vi "RT FIFO Variables - local.vi"() -> ()   [LabVIEW 2017]
doc: "Uses RT FIFO-enabled shared variables to communicate data between loops of different priorities without impacting determinism."
uses:
  <vilib>/Platform/TimedLoop/XDataNode/timing_clust.ctl
  <vilib>/Platform/TimedLoop/XDataNode/nitl_modes.ctl
  <vilib>/Platform/TimedLoop/XDataNode/wakeup.ctl
  <vilib>/platform/TimedLoop/XDataNode/XDataNode.xnode
  <vilib>/Platform/TimedLoop/XDataNode/XDNodeRunTimeDep.lvlib
panel:
  in  "Amplitude":dbl(slide)=5.0 scale=0.0..10.0
  in  "Stop":bool
  out "Result Data":dbl(graph)
  # "Overview: Uses RT FIFO-enabled shared variables to communicate data between loops of different priorities without impacting determinism.\nRequirements: LabVIEW Real-Time Module\nInstructions:\n1. In Measurement & Automation Explorer, ensure that LabVIEW Real-Time and the Network Variable Engine are installed on your RT target.\n2. From the Project Explorer window, set the IP address of your RT target.\n3. Run the VI.\n4. Adjust the Amplitude slider, which will update Result Data chart. \n5. Click the Stop button."
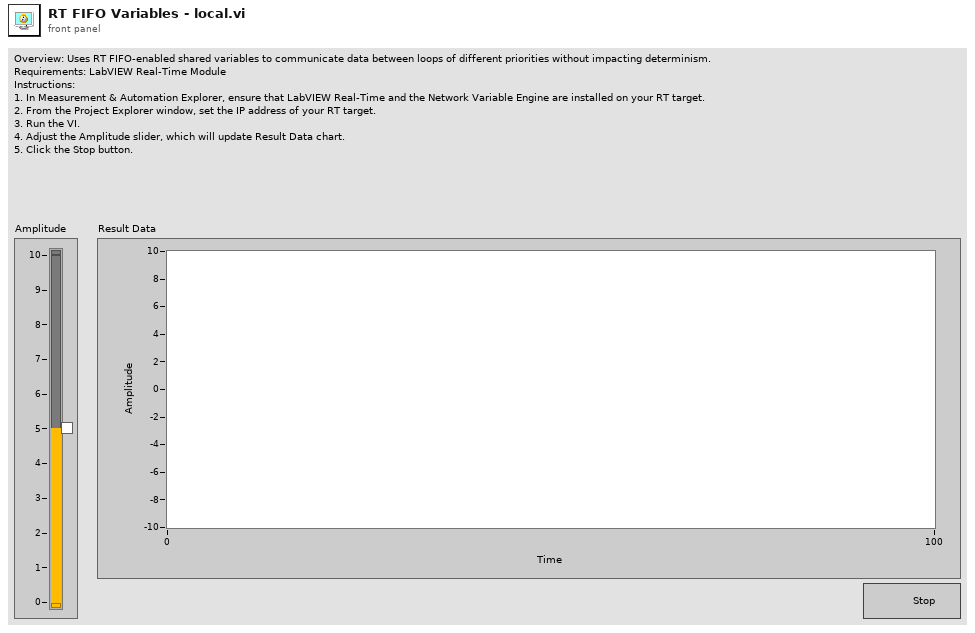
[diagram p1: front panel]
types:
  T1 = typedef "XDNodeRunTimeDep.lvlib/timing_clust.ctl" = cluster{"Expected End [f-1]":u64, "Actual End [f-1]":u64, "Finished Late? [f-1]":bool, "Expected End [i-1]":u64, "Actual End [i-1]":u64, "Finished Late? [i-1]":bool, "Expected Start [i]":u64, "Actual Start [i]":u64, "Expected Start [f]":u64, "Actual Start [f]":u64, "Source Name":string, "Structure Name":string, "Period":i64, "Deadline":i64, "Offset":i64, "Start":i64, "Priority":i32, "Timeout":i32, "Mode":T2, "Wakeup Reason":T3, "Error":errorcluster, "Source Type":string, "Secondary Source Type":string, "Global End Time":u64, "Global Start Time":u64, "Frame Duration":u64, "Iteration Duration":u64, "Assigned CPU":i32, "I/O Scan Engine Mode":u32}
  T2 = typedef "XDNodeRunTimeDep.lvlib/nitl_modes.ctl" = enum32{"No Change", "Process missed periods, maintain original phase", "Discard missed periods, maintain original phase", "Process missed periods, ignore original phase", "Discard missed periods, ignore original phase"}
  T3 = typedef "XDNodeRunTimeDep.lvlib/wakeup.ctl" = enum32{"Normal", "Aborted", "Asynchronous wakeup", "Timing source error", "Timed loop error", "Timeout"}
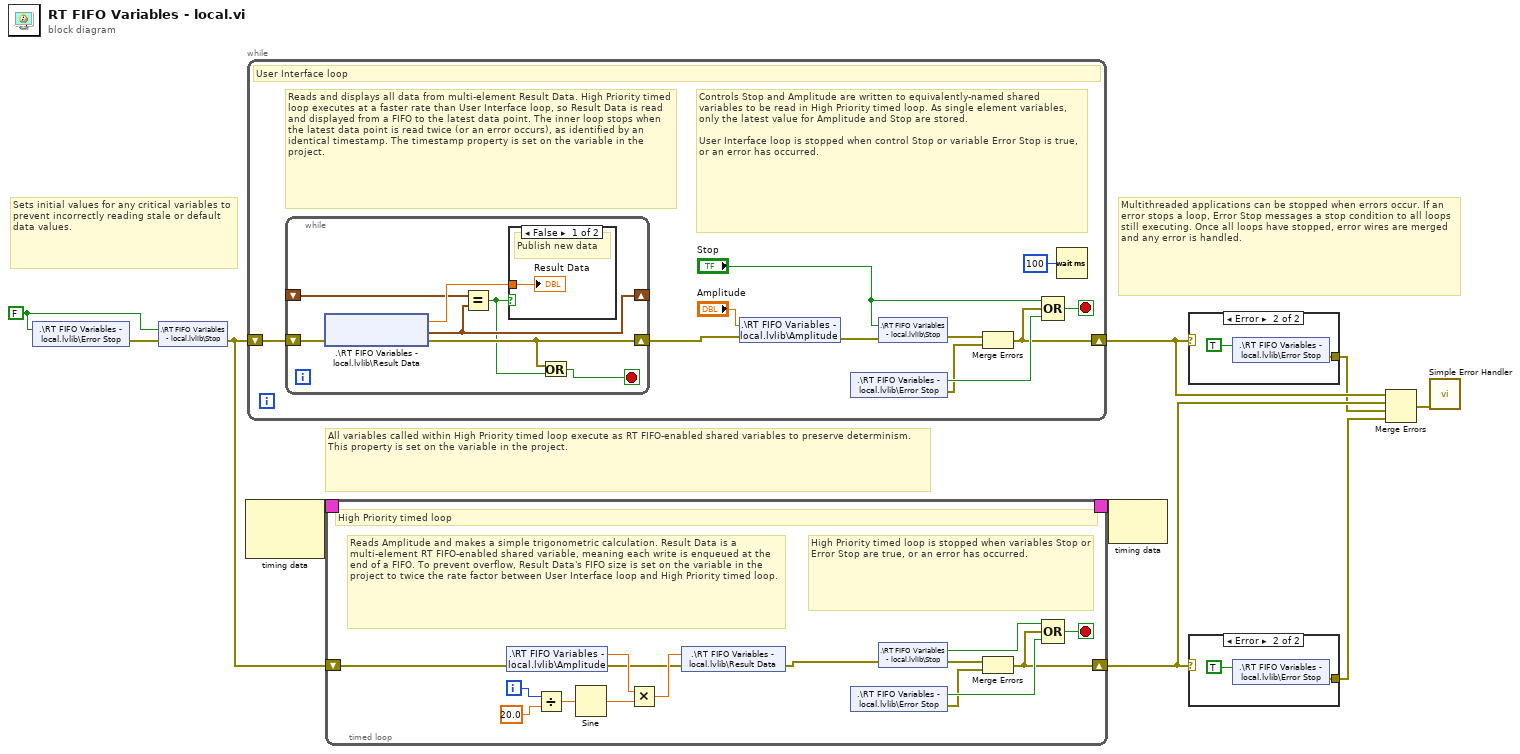
[diagram p0: block diagram]
diagram:
  w6 = FALSE ("Stop")
  # "All variables called within High Priority timed loop execute as RT FIFO-enabled shared variables to preserve determinism. This property is set on the variable in the project."
  # "Multithreaded applications can be stopped when errors occur. If an error stops a loop, Error Stop messages a stop condition to all loops still executing. Once all loops have stopped, error wires are merged and any error is handled."
  # "Sets initial values for any critical variables to prevent incorrectly reading stale or default data values."
  n1 = shared-variable ".\\RT FIFO Variables - local.lvlib\\Error Stop"(w6) -> (error out=w7:errorcluster)  [unwired: 1 in]
  n2 = shared-variable ".\\RT FIFO Variables - local.lvlib\\Stop"(w6, error in=w7) -> (error out=w8:errorcluster)
  n3 = node-c288() -> (w10:T1)  [unwired: 1 in, 1 out]
  n4 = while "User Interface loop" {
    shift-right: [w12] -> w4
    shift-left: w8 -> [w20]
    stop <- w21 stop-if-true
    # "Controls Stop and Amplitude are written to equivalently-named shared variables to be read in High Priority timed loop. As single element variables, only the latest value for Amplitude and Stop are stored.\n\nUser Interface loop is stopped when control Stop or variable Error Stop is true, or an error has occurred."
    # "Reads and displays all data from multi-element Result Data. High Priority timed loop executes at a faster rate than User Interface loop, so Result Data is read and displayed from a FIFO to the latest data point. The inner loop stops when the latest data point is read twice (or an error occurs), as identified by an identical timestamp. The timestamp property is set on the variable in the project."
    # "User Interface loop"
    n5 = while {
      shift-right: [w26] -> _
      shift-left: _ -> [w25]
      shift-right: [w24] -> w18
      shift-left: w20 -> [w28]
      stop <- w22 stop-if-true
      n6 = shared-variable ".\\RT FIFO Variables - local.lvlib\\Result Data"(error in=w28) -> (w27:dbl, error out=w24:errorcluster, w26:timestamp)
      n7 = Equal?(x=w25, y=w26) -> (x = y?=w23:bool)
      n8 = case shown="False" w23 {
        tunnel: w27 -> [w29 _]
        frame False {
          # "Publish new data"
          "Result Data" <- w29
        }
        frame True {
          # "No new data"
        }
      }
      n9 = Or(x=w24, y=w23) -> (x .or. y?=w22:bool)
    }
    n10 = shared-variable ".\\RT FIFO Variables - local.lvlib\\Amplitude"("Amplitude", error in=w18) -> (error out=w19:errorcluster)
    n11 = shared-variable ".\\RT FIFO Variables - local.lvlib\\Error Stop"() -> (w14:bool, error out=w11:errorcluster)  [unwired: 1 in]
    n12 = shared-variable ".\\RT FIFO Variables - local.lvlib\\Stop"("Stop", error in=w19) -> (error out=w13:errorcluster)
    n13 = Merge Errors(w13, w11) -> (w12:errorcluster)
    n14 = Compound Arithmetic op=OR("Stop", w12, w14) -> (w21:bool)
    n15 = Wait (ms)(milliseconds to wait=u32 100 ("millisecond multiple")) -> ()  [unwired: 1 out]
  }
  n16 = timed-loop "High Priority timed loop" {
    timing: w10 -> [_]
    timing-out: [_] -> w9
    shift-right: [w31] -> w2
    shift-left: w8 -> [w35]
    i -> [w40]
    stop <- w44 stop-if-true
    # "Reads Amplitude and makes a simple trigonometric calculation. Result Data is a multi-element RT FIFO-enabled shared variable, meaning each write is enqueued at the end of a FIFO. To prevent overflow, Result Data's FIFO size is set on the variable in the project to twice the rate factor between User Interface loop and High Priority timed loop."
    # "High Priority timed loop is stopped when variables Stop or Error Stop are true, or an error has occurred."
    # "High Priority timed loop"
    n17 = shared-variable ".\\RT FIFO Variables - local.lvlib\\Amplitude"(error in=w35) -> (w38:dbl, error out=w36:errorcluster)
    n18 = Divide(x=w40, y=20.0) -> (x/y=w42:dbl)
    n19 = Sine(x=w42) -> (sin(x)=w41:dbl)
    n20 = Multiply(x=w38, y=w41) -> (x*y=w37:dbl)
    n21 = shared-variable ".\\RT FIFO Variables - local.lvlib\\Result Data"(w37, error in=w36) -> (error out=w34:errorcluster)
    n22 = shared-variable ".\\RT FIFO Variables - local.lvlib\\Error Stop"() -> (w33:bool, error out=w30:errorcluster)  [unwired: 1 in]
    n23 = shared-variable ".\\RT FIFO Variables - local.lvlib\\Stop"(error in=w34) -> (w39:bool, error out=w32:errorcluster)
    n24 = Merge Errors(w32, w30) -> (w31:errorcluster)
    n25 = Compound Arithmetic op=OR(w39, w31, w33) -> (w44:bool)
  }
  n26 = node-c288(w9) -> ()  [unwired: 1 out]
  n27 = case shown="Error" w4 {
    tunnel: [_ w47] -> w1
    frame No Error {
    }
    frame Error {
      n28 = shared-variable ".\\RT FIFO Variables - local.lvlib\\Error Stop"(TRUE ("Error Stop")) -> (error out=w47:errorcluster)  [unwired: 1 in]
    }
  }
  n29 = case shown="Error" w2 {
    tunnel: [_ w49] -> w3
    frame No Error {
    }
    frame Error {
      n30 = shared-variable ".\\RT FIFO Variables - local.lvlib\\Error Stop"(TRUE ("Error Stop")) -> (error out=w49:errorcluster)  [unwired: 1 in]
    }
  }
  n31 = Merge Errors(w4, w2, w1, w3) -> (w5:errorcluster)
  n32 = call <vilib>:"Simple Error Handler.vi"("error in (no error)"=w5) -> ()  [unwired: 4 in, 5 out]
